vi "Get Program Status.vi"(8 "error in (no error)":errorcluster, 11 "ARS-0220 in":refnum<class "ARS-0220.lvclass">) -> (0 "error out":errorcluster, 2 "Program State":T1 {"remaining time" format="%<%H:%M>t"}, 3 "ARS-0220 out":refnum<class "ARS-0220.lvclass">)   [LabVIEW 2021, in "Environment Chamber.lvlib" / "ARS-0220.lvclass"]
uses:
  ARS-0220.lvclass
  Support Libraries/Climatic Chamber/Private/Type Defs/Program OpState Cluster.ctl
  ARS-0220.lvclass/ARS-0220.ctl
  Support Libraries/Climatic Chamber/Climatic Chamber.lvlib
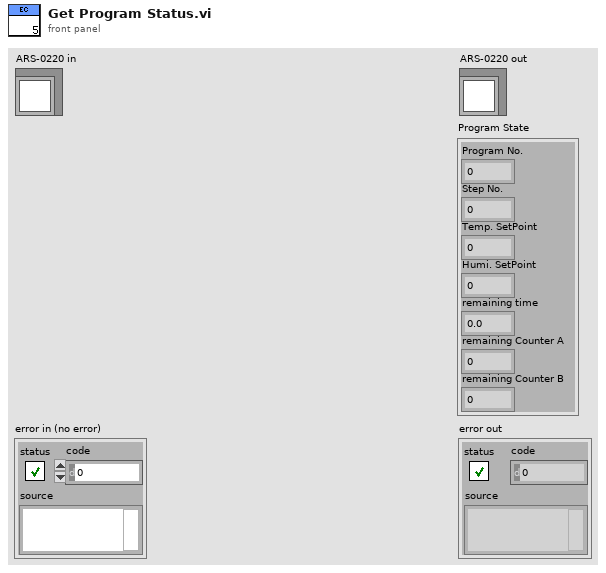
[diagram p1: front panel]
types:
  T1 = typedef "Environment Chamber.lvlib/Climatic Chamber.lvlib/Program OpState Cluster.ctl" = cluster{"Program No.":i32, "Step No.":i32, "Temp. SetPoint":dbl, "Humi. SetPoint":dbl, "remaining time":dbl, "remaining Counter A":i32, "remaining Counter B":i32}
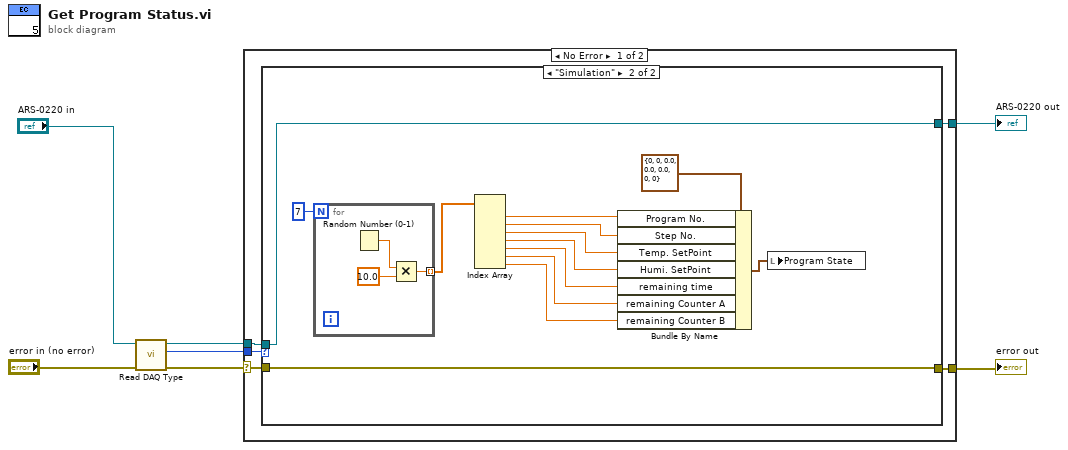
[diagram p0: block diagram]
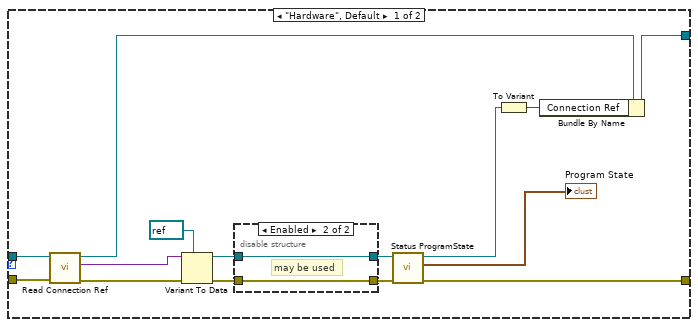
[diagram p2: hidden frame]
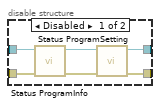
[diagram p3: hidden frame]
diagram:
  n1 = call "Read DAQ Type.vi"("error in (no error)"="error in (no error)", "ARS-0220 in"="ARS-0220 in") -> ("error out"=w6:errorcluster, "DAQ Type"=w4:enum16{"Hardware", "Simulation"}, "ARS-0220 out"=w3:refnum<class "ARS-0220.lvclass">)  [unwired: 7 in]
  n2 = case shown="No Error" w6 {
    selector: w6 -> [w10 w52]
    tunnel: w4 -> [w12 _]
    tunnel: w3 -> [w11 w53]
    tunnel: [w9 w52] -> w2
    tunnel: [w8 w53] -> w1
    frame No Error {
      n3 = case shown="\"Simulation\"" w12 {
        tunnel: w11 -> [w27 w48]
        tunnel: w10 -> [w26 w47]
        tunnel: [w20 w47] -> w9
        tunnel: [w18 w48] -> w8
        frame "Hardware", Default {
          n4 = call "Read Connection Ref.vi"("error in (no error)"=w26, "ARS-0220 in"=w27) -> ("error out"=w23:errorcluster, "Connection Ref"=w24:variant, "ARS-0220 out"=w19:refnum<class "ARS-0220.lvclass">)  [unwired: 7 in]
          n5 = Variant To Data(error in=w23, type=refnum<visa-resource-name> refnum ("VISA resource name"), Variant=w24) -> (data=w15:refnum<visa-resource-name>, error out=w22:errorcluster)
          n6 = disable-structure shown="Enabled" {
            disable-tunnel: w22 -> [w33 w34]
            disable-tunnel: [w31 w34] -> w21
            disable-tunnel: w15 -> [w30 w35]
            disable-tunnel: [w28 w35] -> w14
            frame Disabled {
              n7 = call "Status ProgramInfo.vi"("error in (no error)"=w33, "VISA resource name"=w30) -> ("error out"=w32:errorcluster, "VISA resource name out"=w29:refnum<visa-resource-name>)  [unwired: 4 in, 4 out]
              n8 = call "Status ProgramSetting.vi"("error in (no error)"=w32, "VISA resource name"=w29) -> ("error out"=w31:errorcluster, "VISA resource name out"=w28:refnum<visa-resource-name>)  [unwired: 5 in, 3 out]
            }
            frame Enabled {
              # "may be used"
            }
          }
          n9 = call "Status ProgramState.vi"("error in (no error)"=w21, "VISA resource name"=w14) -> ("error out"=w20:errorcluster, "Program State"=→"Program State":T1, "VISA resource name out"=w16:refnum<visa-resource-name>)  [unwired: 7 in]
          n10 = To Variant(anything=w16) -> (Variant=w17:variant)
          n11 = Bundle By Name(cluster=w19, "Connection Ref"=w17) -> (w18:refnum<class "ARS-0220.lvclass">)
        }
        frame "Simulation" {
          n12 = for {
            N: 7 -> [_]
            tunnel: [w49] -> w44 mode=indexing
            n13 = Random Number (0-1)() -> (number: 0 to 1=w51:dbl)
            n14 = Multiply(x=w51, y=10.0) -> (x*y=w49:dbl)
          }
          n15 = Index Array(array=w44) -> (element #1=w43:dbl, element #2=w42:dbl, element #3=w41:dbl, element #4=w40:dbl, element #5=w39:dbl, element #6=w38:dbl, element #7=w37:dbl)  [unwired: 7 in]
          n16 = Bundle By Name(cluster=T1 {"Program No."=0, "Step No."=0, "Temp. SetPoint"=0.0, "Humi. SetPoint"=0.0, "remaining time"=0.0, "remaining Counter A"=0, "remaining Counter B"=0} ("Program State"), "Program No."=w43, "Step No."=w42, "Temp. SetPoint"=w41, "Humi. SetPoint"=w40, "remaining time"=w39, "remaining Counter A"=w38, "remaining Counter B"=w37) -> (w36:T1)
          n17 = local write "Program State"(w36) -> ()
        }
      }
    }
    frame Error {
    }
  }
  "error out" <- w2
  "ARS-0220 out" <- w1
